vi "SubPanelTypecast.vi"(0 "Ctl Refnum":refnum<vi>, 7 "Control Path In":string[](array[string]), 11 "Error In":errorcluster) -> (4 "Controls[]":refnum<vi>[](array[refnum]), 8 "Control Path Out":string[](array[string]), 15 "Error Out":errorcluster)   [LabVIEW 2016]
doc: "This VI gives the reference of controls present inside the inserted VI of the SubPanel"
uses:
  <vilib>/Utility/error.llb/Error Cluster From Error Code.vi
  <vilib>/ErrorRing/Error Ring.xnode
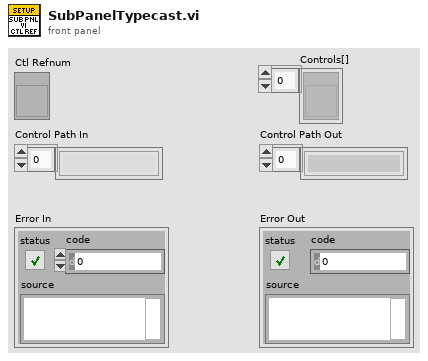
[diagram p1: front panel]
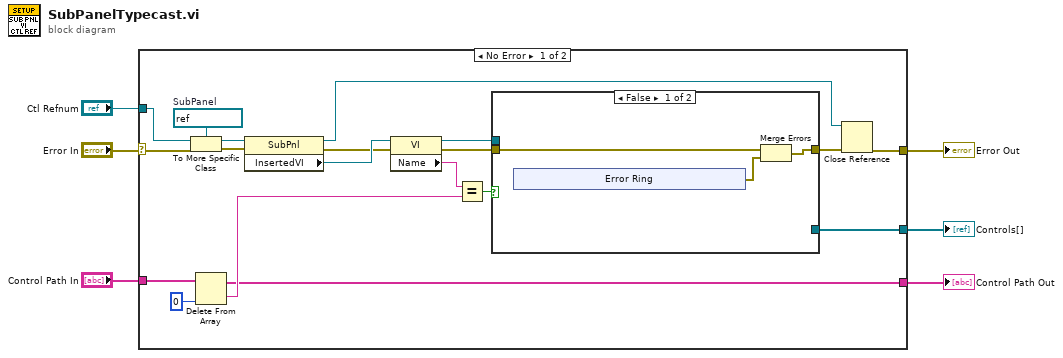
[diagram p0: block diagram]
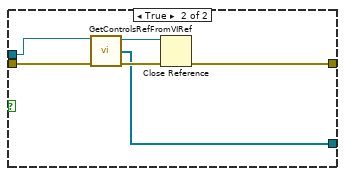
[diagram p2: hidden frame]
diagram:
  n1 = case shown="No Error" "Error In" {
    selector: "Error In" -> [w12 w41]
    tunnel: "Control Path In" -> [w25 w40]
    tunnel: "Ctl Refnum" -> [w24 _]
    tunnel: [w15 _] -> w4
    tunnel: [w14 w40] -> w3
    tunnel: [w13 w41] -> w2
    frame No Error {
      w21 = refnum<vi> refnum  # SubPanel
      n2 = To More Specific Class(target class=w21, reference=w24, error in=w12) -> (specific class reference=w23:refnum<vi>, error out=w22:errorcluster)
      n3 = Delete From Array(array=w25, index=0) -> (deleted portion=w16:string, array with subset deleted=w14:string[])  [unwired: 1 in]
      n4 = property class="SubPnl"(reference=w23, error in=w22) -> (reference out=w18:refnum<vi>, error out=w19:errorcluster, "InsertedVI"=w20:refnum<vi>)
      n5 = property class="VI"(reference=w20, error in=w19) -> (reference out=w8:refnum<vi>, error out=w9:errorcluster, "Name"=w11:string)
      n6 = Equal?(x=w11, y=w16) -> (x = y?=w10:bool)
      n7 = case shown="False" w10 {
        tunnel: w9 -> [w28 w38]
        tunnel: [w27 w35] -> w7
        tunnel: w8 -> [_ w39]
        tunnel: [_ w36] -> w15
        frame False {
          n8 = xnode "Error Ring"() -> ("error out"=w26:errorcluster)
          n9 = Merge Errors(w28, w26) -> (w27:errorcluster)
        }
        frame True {
          n10 = call "GetControlsRefFromVIRef.vi"("VI Reference In"=w39, "Error In"=w38) -> ("VI Reference Out"=w34:refnum<vi>, "Controls[]"=w36:refnum<vi>[], "Error Out"=w37:errorcluster)  [unwired: 11 in]
          n11 = Close Reference(reference=w34, error in (no error)=w37) -> (error out=w35:errorcluster)
        }
      }
      n12 = Close Reference(reference=w18, error in (no error)=w7) -> (error out=w13:errorcluster)
    }
    frame Error {
    }
  }
  "Controls[]" <- w4
  "Control Path Out" <- w3
  "Error Out" <- w2
